vi "PCO_SetCoolingSetpointTemperature.vi"(8 "error in (no error)":errorcluster {"code" format="%x"}, 10 "sCoolSet":i16, 11 "ph":u64) -> (0 "error out":errorcluster {"code" format="%x"}, 2 "ErrorMessage":i32 format="%x", 3 "ph out":u64)   [LabVIEW 2019, in "SDK.lvlib" / "ImageSensor.lvlib"]
doc: "<b>Description:</b>\nThis function does set the temperature setpoint for the image sensor in °C. A peltier cooling unit is used to regulate the temperature of the sensor to the given temperature setpoint. Thus reduces dark current noise and improves image quality. Valid values for the setpoint must be in the range between sMinCoolSetDESC and sMaxCoolSetDESC. The current temperature must be checked to see when the setpoint temperature is reached.\n\nDefault temperature regulation setpoint is defined in sDefaultCoolSetDESC parameter of the PCO_Description structure. Temperature regulation for the sensor is not available, when both temperature range parameters sMinCoolSetDESC and sMaxCoolSetDESC of the PCO_Description structure are zero.\n\nValid range depends on camera type. Invalid values result in a failure response message.\nThe current temperature of the sensor can be read out with the PCO_GetTemperature command.\n\n<b>Supported camera type:</b>\npco.1300, pco.1600, pco.2000, pco.4000, pco.edge, pco.flim\n\n<b>Descriptor dependency:</b>\nsMinCoolSetDESC,sMaxCoolSetDESC\ndwGeneralCapsDESC1: COOLING_SETPOINTS"
uses:
  ImageSensor.lvlib
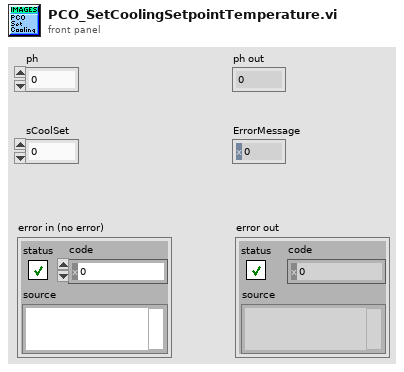
[diagram p1: front panel]
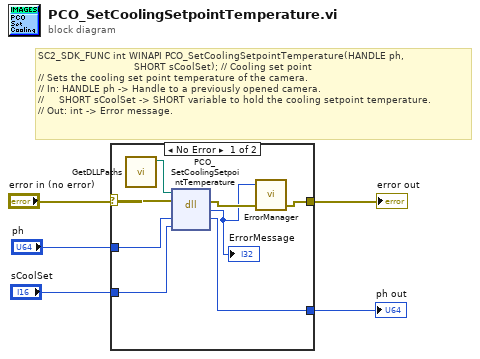
[diagram p0: block diagram]
diagram:
  # "SC2_SDK_FUNC int WINAPI PCO_SetCoolingSetpointTemperature(HANDLE ph,\n                                SHORT sCoolSet); // Cooling set point\n// Sets the cooling set point temperature of the camera.\n// In: HANDLE ph -> Handle to a previously opened camera.\n//     SHORT sCoolSet -> SHORT variable to hold the cooling setpoint temperature.\n// Out: int -> Error message."
  n1 = case shown="No Error" "error in (no error)" {
    selector: "error in (no error)" -> [w10 w15]
    tunnel: "ph" -> [w13 w14]
    tunnel: [w12 w14] -> w4
    tunnel: "sCoolSet" -> [w11 _]
    tunnel: [w8 w15] -> w2
    frame No Error {
      n2 = call "GetDLLPaths.vi"() -> ("SC2_Cam_Path"=w6:path)  [unwired: 9 in, 2 out]
      n3 = dll-call lib="?" fn="PCO_SetCoolingSetpointTemperature"(path in=w6, error in=w10, "ph"=w13, "sCoolSet"=w11) -> (error out=w9:errorcluster, "return type"=w7:i32, "ph"=w12:u64)  [unwired: 2 in, 1 out]
      "ErrorMessage" <- w7
      n4 = call "ErrorManager.vi"("error in (no error)"=w9, "error code"=w7) -> ("error out"=w8:errorcluster)  [unwired: 3 in]
    }
    frame Error {
    }
  }
  "ph out" <- w4
  "error out" <- w2
